vi "Absolute Angle Difference in Radians.vi"(9 "angle 2 (rad)":dbl, 11 "angle 1 (rad)":dbl) -> (2 "|angle 1 - angle 2| (rad)":dbl)   [LabVIEW 2017, in "NI_Robotics Utilities.lvlib"]
doc: "This VI is deprecated. Use <vi.lib>\\Analysis\\coordinate.llb\\Absolute Angle Difference.vi instead."
uses:
  <vilib>/robotics/Utilities/NI_Robotics Utilities.lvlib
  <vilib>/robotics/Utilities/Angle Range_Radians.ctl
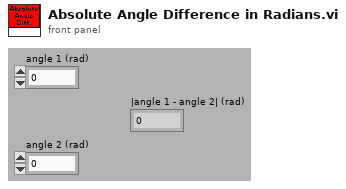
[diagram p1: front panel]
types:
  T1 = typedef "NI_Robotics Utilities.lvlib/Angle Range_Radians.ctl" = enum16{"none", "-pi to pi", "0 to 2*pi"}
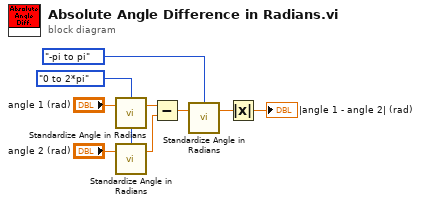
[diagram p0: block diagram]
diagram:
  w2 = Angle_Range_Radians."0 to 2*pi" ("range (-pi to pi)")
  n1 = call <vilib>:"Standardize Angle in Radians.vi"("angle in (rad)"="angle 1 (rad)", "range (-pi to pi)"=w2) -> ("angle out (rad)"=w7:dbl)  [unwired: 3 in]
  n2 = call <vilib>:"Standardize Angle in Radians.vi"("angle in (rad)"="angle 2 (rad)", "range (-pi to pi)"=w2) -> ("angle out (rad)"=w6:dbl)  [unwired: 3 in]
  n3 = Subtract(x=w7, y=w6) -> (x-y=w5:dbl)
  n4 = call <vilib>:"Standardize Angle in Radians.vi"("angle in (rad)"=w5, "range (-pi to pi)"=Angle_Range_Radians."-pi to pi") -> ("angle out (rad)"=w4:dbl)  [unwired: 3 in]
  n5 = Absolute Value(x=w4) -> (abs(x)=→"|angle 1 - angle 2| (rad)":dbl)
